vi "Configure Valve.vi"(8 "error in (no error)":errorcluster, 9 "External Valve Number (1:1)":u16(ring)=1 items=["1"=1, "2"=2, "3"=3, "4"=4, "6"=6, "7"=7, "8"=8], 10 "Enable External Solenoid Valve (Enable)":bool=TRUE, 11 "VISA resource name":refnum<visa-resource-name>) -> (0 "error out":errorcluster, 3 "VISA resource name out":refnum<visa-resource-name>)   [LabVIEW 2023, in "Fluke Molbox 1 Plus.lvlib"]
doc: "Sets the status of an external solenoid valve. The molbox1+ has the option of controlling up to eight external valves."
uses:
  Fluke Molbox 1 Plus.lvlib
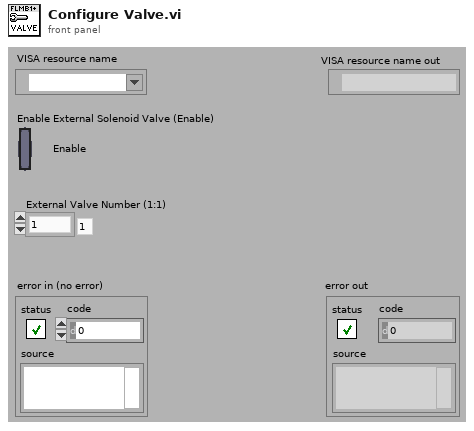
[diagram p1: front panel]
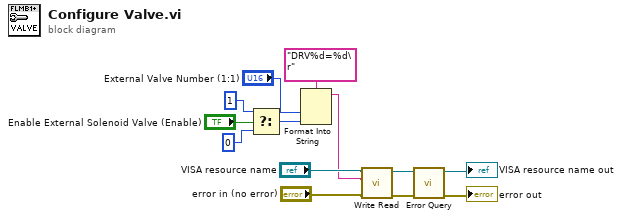
[diagram p0: block diagram]
diagram:
  n1 = Select(t=1, s="Enable External Solenoid Valve (Enable)", f=0) -> (s? t:f=w9:i32)
  n2 = Format Into String(format string="DRV%d=%d\r", "External Valve Number (1:1)", w9) -> (resulting string=w5:string)  [unwired: 2 in, 1 out]
  n3 = call "Write Read.vi"("error in (no error)"="error in (no error)", "Write String"=w5, "VISA resource name"="VISA resource name") -> ("error out"=w3:errorcluster, "VISA resource name out"=w4:refnum<visa-resource-name>)  [unwired: 6 in, 1 out]
  n4 = call "Error Query.vi"("error in (no error)"=w3, "VISA resource name"=w4) -> ("error out"=→"error out":errorcluster, "VISA resource name out"=→"VISA resource name out":refnum<visa-resource-name>)  [unwired: 6 in, 2 out]
